vi "onDestroy.vi"(8 "error in (no error)":errorcluster, 11 "CircularBuffer":refnum<class "CircularBuffer.lvclass">) -> (0 "error out":errorcluster, 3 "CircularBuffer out":refnum<class "CircularBuffer.lvclass">)   [LabVIEW 2016, in "CircularBuffer.lvclass"]
doc: "JKI State Machine Objects (SMO) 1.0.4.18\nJKI - JKI\nCopyright (c) 2016, JKI"
uses:
  CircularBuffer.lvclass
  <vilib>/JKI/JKI SMO/SMO/SMO.lvclass
  types/type/type.lvclass
panel:
  # "For instructions on how to use the JKI State Machine Objects, examples and video tutorials, visit:\nhttp://jki.net/state-machine-objects/\n\nJKI State Machine Objects™\nhttp://jki.net/state-machine-objects/\nCopyright (C) 2005-2015, JKI <info@jki.net>\nALL RIGHTS RESERVED"
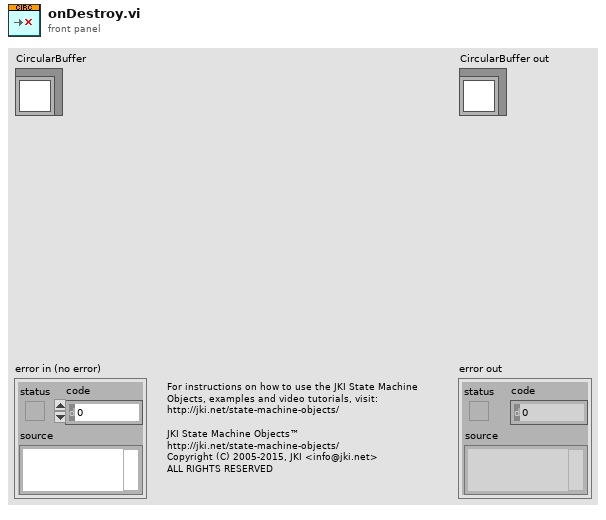
[diagram p1: front panel]
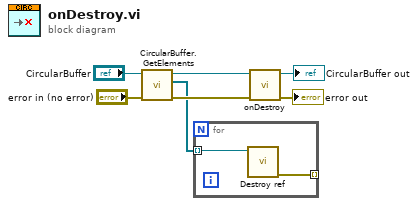
[diagram p0: block diagram]
diagram:
  n1 = call "CircularBuffer.GetElements.vi"("error in (no error)"="error in (no error)", "CircularBuffer in"="CircularBuffer") -> ("error out"=w2:errorcluster, "Elements"=w1:refnum<data-value>[], "CircularBuffer out"=w4:refnum<class "CircularBuffer.lvclass">)  [unwired: 7 in]
  n2 = for {
    tunnel: w1 -> [w9] mode=indexing
    tunnel: [w8] -> _ mode=indexing
    n3 = call "Destroy ref.vi"("data value reference"=w9) -> ("error out"=w8:errorcluster)  [unwired: 10 in]
  }
  n4 = call-parent "onDestroy.vi"("error in (no error)"=w2, "SMO"=w4) -> ("error out"=→"error out":errorcluster, "SMO out"=→"CircularBuffer out":refnum<class "CircularBuffer.lvclass">)  [unwired: 8 in]
